vi "Populate TX PDO Mapping.vi"(8 "error in":errorcluster, 11 "UI Actor in":refnum<class "UI Actor.lvclass">) -> (0 "error out":errorcluster, 3 "UI Actor out":refnum<class "UI Actor.lvclass">)   [LabVIEW 2020, in "UI Actor.lvlib" / "UI Actor.lvclass"]
uses:
  UI Actor.lvclass
  UI Actor.lvclass/UI Actor.ctl
  PDO Slot/PDO Slot.lvclass
  Electronic Datasheet/Electronic Datasheet.lvclass
  PDO Grid/PDO Grid.lvclass
  Core/OD Entry/OD Entry.lvclass
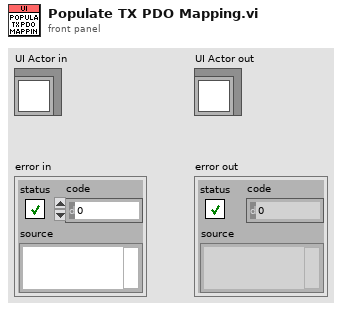
[diagram p1: front panel]
types:
  T1 = map{path, refnum<class "Electronic Datasheet.lvclass">}
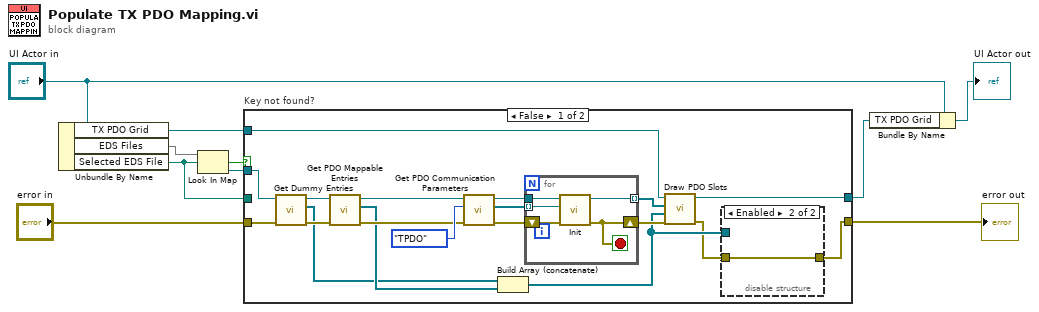
[diagram p0: block diagram]
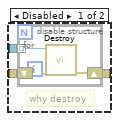
[diagram p2: hidden frame]
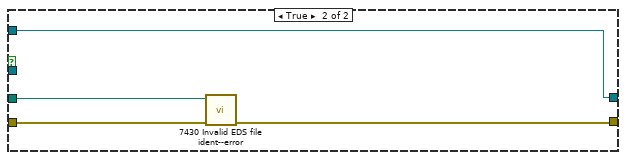
[diagram p3: hidden frame]
diagram:
  n1 = Unbundle By Name("UI Actor in") -> ("TX PDO Grid"=w3:refnum<class "PDO Grid.lvclass">, "EDS Files"=w9:T1, "Selected EDS File"=w6:path)
  n2 = Look In Map(map=w9, key=w6) -> (key not found?=w8:bool, value=w5:refnum<class "Electronic Datasheet.lvclass">)  [unwired: 1 in]
  n3 = case "Key not found?" shown="False" w8 {
    tunnel: "error in" -> [w25 w45]
    tunnel: w6 -> [_ w44]
    tunnel: w5 -> [w19 _]
    tunnel: w3 -> [w22 w43]
    tunnel: [w11 w42] -> w2
    tunnel: [w23 w43] -> w1
    frame False {
      n4 = call "Get Dummy Entries.vi"("Error In"=w25, "reference in"=w19) -> ("Error Out"=w20:errorcluster, "Dummy Entries"=w14:refnum<class "OD Entry.lvclass">[], "reference out"=w17:refnum<class "Electronic Datasheet.lvclass">)  [unwired: 7 in]
      n5 = call "Get PDO Mappable Entries.vi"("error in"=w20, "Electronic Datasheet in"=w17) -> ("error out"=w18:errorcluster, "PDO Mappable Entries"=w15:refnum<class "OD Entry.lvclass">[], "Electronic Datasheet out"=w16:refnum<class "Electronic Datasheet.lvclass">)  [unwired: 7 in]
      n6 = call "Get PDO Communication Parameters.vi"("error in"=w18, "Type"=enum16{"TPDO", "RPDO"}."TPDO", "EDS in"=w16) -> ("error out"=w28:errorcluster, "Entries"=w27:refnum<class "OD Entry.lvclass">[], "EDS out"=w26:refnum<class "Electronic Datasheet.lvclass">)  [unwired: 6 in]
      n7 = Build Array (concatenate)(w14, w15) -> (w13:refnum<class "OD Entry.lvclass">[])
      n8 = for {
        shift-right: [w37] -> w24
        shift-left: w28 -> [w41]
        tunnel: w27 -> [w40] mode=indexing
        tunnel: [w39] -> w21 mode=indexing
        tunnel: w26 -> [w38]
        stop <- w37 stop-if-true
        n9 = call "Init.vi"("error in"=w41, "PDO Communication Parameter Entry"=w40, "Electronic Datasheet"=w38) -> ("error out"=w37:errorcluster, "PDO Slot out"=w39:refnum<class "PDO Slot.lvclass">)  [unwired: 7 in]
      }
      n10 = call-dynamic "Draw PDO Slots.vi"("error in"=w24, "PDO Mappable Entries"=w13, "PDO Slots"=w21, "PDO Grid in"=w22) -> ("error out"=w12:errorcluster, "PDO Grid out"=w23:refnum<class "PDO Grid.lvclass">)  [unwired: 6 in]
      n11 = disable-structure shown="Enabled" {
        disable-tunnel: w13 -> [w32 _]
        disable-tunnel: w12 -> [w31 w36]
        disable-tunnel: [w30 w36] -> w11
        frame Disabled {
          # "why destroy"
          n12 = for {
            shift-right: [w33] -> w30
            shift-left: w31 -> [w34]
            tunnel: w32 -> [w35] mode=indexing
            n13 = call-dynamic "Destroy.vi"("Error In"=w34, "reference in"=w35) -> ("Error Out"=w33:errorcluster)  [unwired: 8 in, 1 out]
          }
        }
        frame Enabled {
        }
      }
    }
    frame True {
      n14 = call "7430 Invalid EDS file ident--error.vi"("error in"=w45, "Selected EDS File"=w44) -> ("error out"=w42:errorcluster)  [unwired: 9 in]
    }
  }
  "error out" <- w2
  n15 = Bundle By Name(cluster="UI Actor in", "TX PDO Grid"=w1) -> (→"UI Actor out":refnum<class "UI Actor.lvclass">)
